vi "Fc_evaluate_state.vi"(8 "error in (no error)":errorcluster, 11 "VI in":refnum<vi>) -> (0 "error out":errorcluster, 2 "Exec.State":T1(ring), 3 "Status out":bool)   [LabVIEW 2022 SP3]
doc: "This function evaluates the execution state of the active window plot."
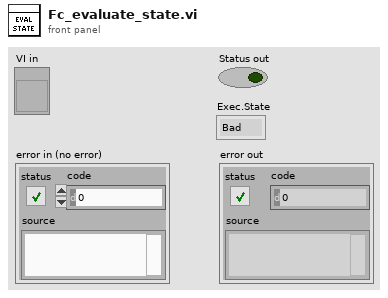
[diagram p1: front panel]
types:
  T1 = enum32{"Bad", "Idle", "Run top level", "Running"}
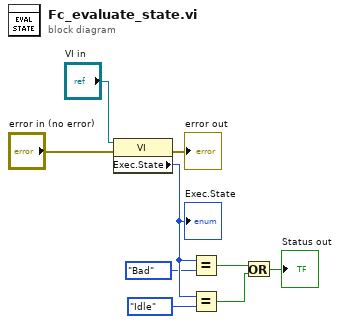
[diagram p0: block diagram]
diagram:
  n1 = property class="VI"(reference="VI in", error in="error in (no error)") -> (error out=→"error out":errorcluster, "Exec.State"=w7:T1)  [unwired: 1 out]
  "Exec.State" <- w7
  n2 = Equal?(x=w7, y=T1."Bad" ("Execution:State")) -> (x = y?=w4:bool)
  n3 = Equal?(x=w7, y=T1."Idle" ("Execution:State")) -> (x = y?=w5:bool)
  n4 = Or(x=w4, y=w5) -> (x .or. y?=→"Status out":bool)
